vi "Write XBoxUSBPort.vi"(8 "error in (no error)":errorcluster, 10 "XBoxUSBPort":T1, 11 "XBoxController in":refnum<class "XBoxController.lvclass">) -> (0 "error out":errorcluster, 3 "XBoxController out":refnum<class "XBoxController.lvclass">)   [LabVIEW 2013, in "XBoxController.lvclass"]
uses:
  XBoxController.lvclass
  <vilib>/Rock Robotics/WPI/Joystick/WPI_JoystickDeviceEnum.ctl
  XBoxController.lvclass/XBoxController.ctl
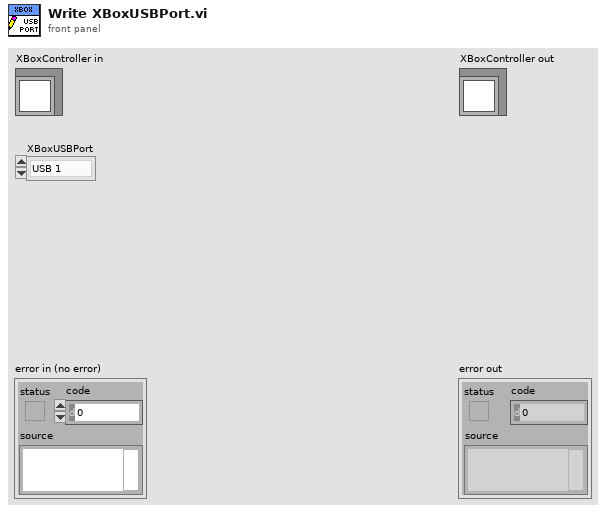
[diagram p1: front panel]
types:
  T1 = typedef "WPI_JoystickDeviceEnum.ctl" = enum16{"USB 1", "USB 2", "USB 3", "USB 4", "Kinect 1", "Kinect 2"}
  T2 = typedef "WPI_JoystickDevRef.ctl" = cluster{"Device":T1}
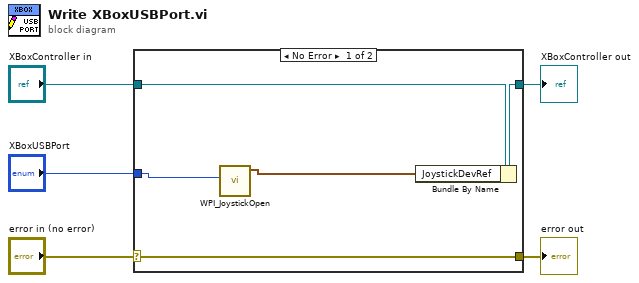
[diagram p0: block diagram]
diagram:
  n1 = case shown="No Error" "error in (no error)" {
    selector: "error in (no error)" -> [w10 w11]
    tunnel: [w10 w11] -> w4
    tunnel: [w8 w12] -> w2
    tunnel: "XBoxController in" -> [w9 w12]
    tunnel: "XBoxUSBPort" -> [w7 _]
    frame No Error {
      n2 = call <vilib>:"WPI_JoystickOpen.vi"("JoystickDevice"=w7) -> ("JoystickDevRef"=w6:T2)  [unwired: 10 in]
      n3 = Bundle By Name(cluster=w9, "JoystickDevRef"=w6) -> (w8:refnum<class "XBoxController.lvclass">)
    }
    frame Error {
    }
  }
  "error out" <- w4
  "XBoxController out" <- w2
